vi "Create Logger.vi"(8 "error in":errorcluster, 10 "Handlers":refnum<class "Handler.lvclass">[](array[class]), 11 "Name":string) -> (0 "error out":errorcluster, 3 "Logger out":refnum<class "Logger.lvclass">)   [LabVIEW 2020, in "hse-logger.lvlib" / "Logger.lvclass"]
doc: "Instantiates a new ``Logger`` object and the specified name and handlers.\n\n____\nHAMPEL SOFTWARE ENGINEERING v2.0.6 (2021-04-15 11:38)"
uses:
  Logger.lvclass
  Handler/Handler.lvclass
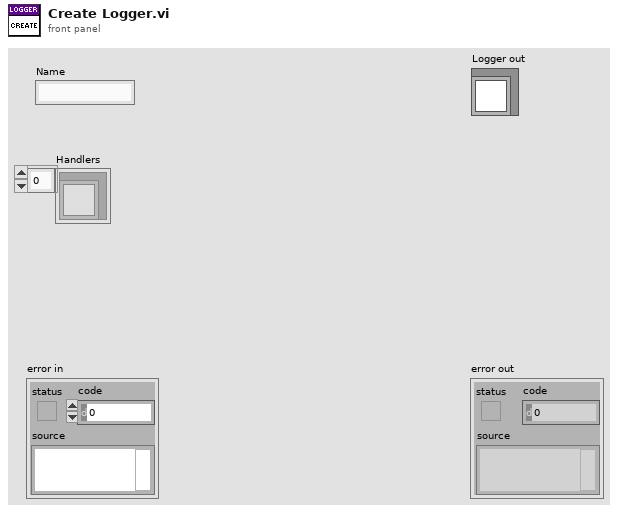
[diagram p1: front panel]
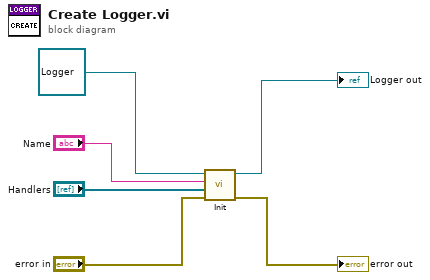
[diagram p0: block diagram]
diagram:
  n1 = call-dynamic "Init.vi"("error in"="error in", "Handlers"="Handlers", "Name"="Name", "Logger in"=refnum<class "Logger.lvclass"> refnum ("hse-logger.lvlib:Logger.lvclass")) -> ("error out"=→"error out":errorcluster, "Logger out"=→"Logger out":refnum<class "Logger.lvclass">)  [unwired: 6 in]
